vi "LogTest1.vi"() -> ()   [LabVIEW 2016]
panel:
  out "Experiment Description 2":T1
  out "date/time string":string
  out "current time":timestamp
  in  "file path":path
  in  "stop":bool
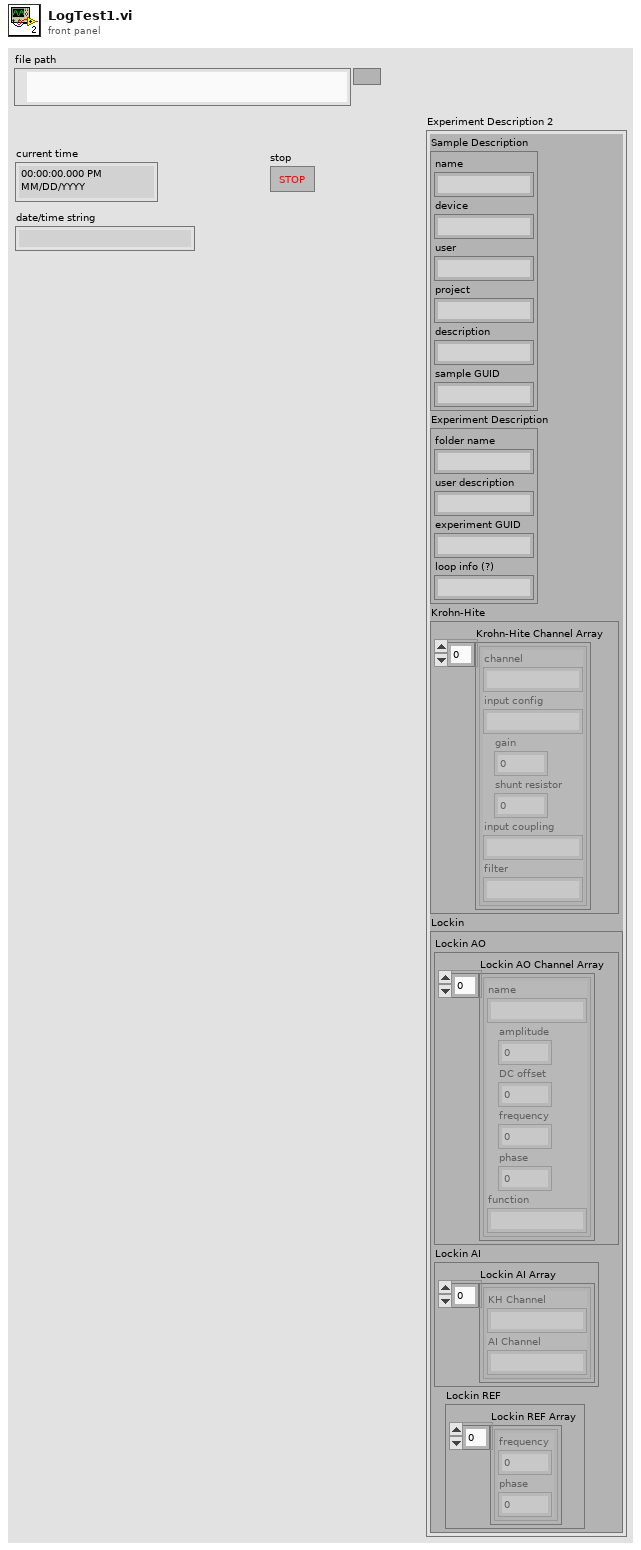
[diagram p1: front panel]
types:
  T1 = cluster{"Sample Description":cluster{"name":string, "device":string, "user":string, "project":string, "description":string, "sample GUID":string}, "Experiment Description":cluster{"folder name":string, "user description":string, "experiment GUID":string, "loop info (?)":string}, "Krohn-Hite":cluster{"Krohn-Hite Channel Array":cluster{"channel":string, "input config":string, "gain":i32, "shunt resistor":i32, "input coupling":string, "filter":string}[]}, "Lockin":cluster{"Lockin AO":cluster{"Lockin AO Channel Array":cluster{"name":string, "amplitude":dbl, "DC offset":dbl, "frequency":dbl, "phase":dbl, "function":string}[]}, "Lockin AI":cluster{"Lockin AI Array":cluster{"KH Channel":string, "AI Channel":string}[]}, "Lockin REF":cluster{"Lockin REF Array":cluster{"frequency":dbl, "phase":dbl}[]}}}
  T2 = enum16{"open", "open or create", "create or replace", "create", "open (read-only)"}
  T3 = cluster{"name":string, "device":string, "user":string, "project":string, "description":string, "sample GUID":string}
  T4 = cluster{"folder name":string, "user description":string, "experiment GUID":string, "loop info (?)":string}
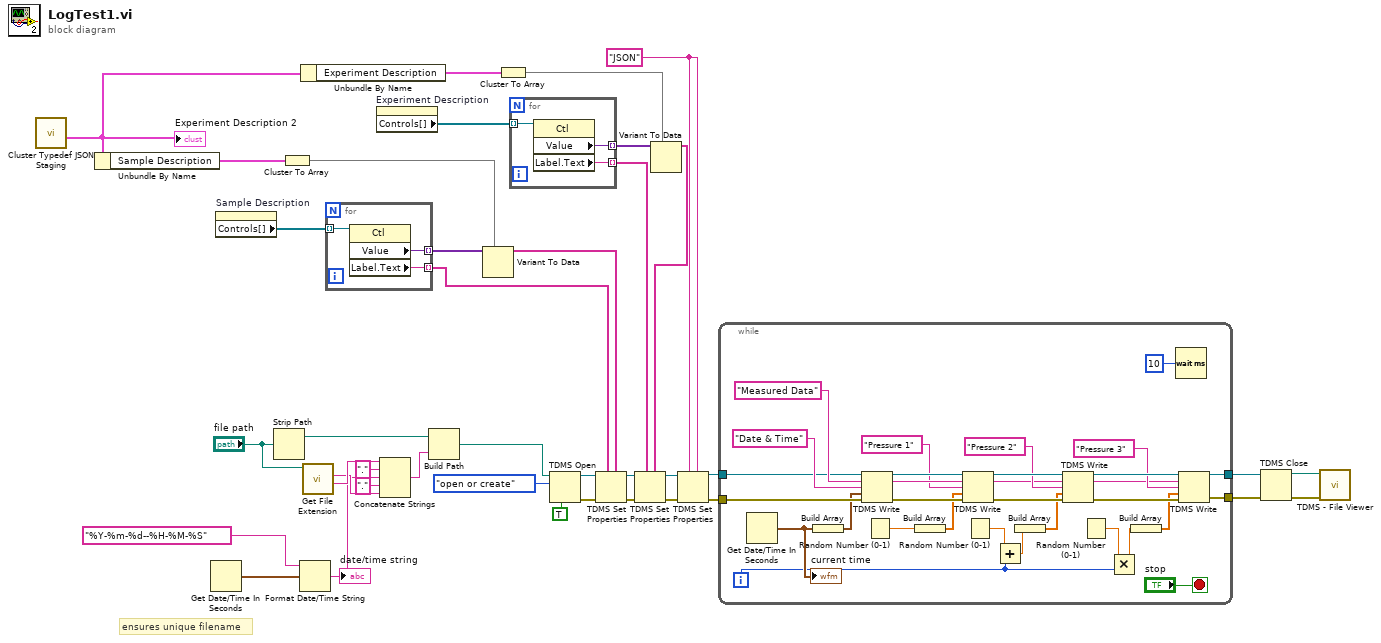
[diagram p0: block diagram]
diagram:
  w1 = "JSON"
  # "ensures unique filename"
  n1 = call "Cluster Typedef JSON Staging.vi"() -> ("Experiment Description 2"=w11:T1)  [unwired: 9 in, 2 out]
  "Experiment Description 2" <- w11
  n2 = Unbundle By Name(w11) -> ("Sample Description"=w16:T3)
  n3 = Get Date/Time In Seconds() -> (seconds since 1Jan1904=w35:timestamp)
  n4 = property on="Sample Description" class="Clust (strict)"() -> ("Controls[]"=w39:refnum<vi>[])  [unwired: 2 in, 2 out]
  n5 = Strip Path(path="file path") -> (stripped path=w19:path)  [unwired: 1 out]
  n6 = Cluster To Array(cluster=w16) -> (array=w37:string[])
  n7 = Format Date/Time String(time format string (%c)="%Y-%m-%d--%H-%M-%S", seconds (now)=w35) -> (date/time string=w31:string)  [unwired: 1 in]
  "date/time string" <- w31
  n8 = Unbundle By Name(w11) -> ("Experiment Description"=w15:T4)
  n9 = call <vilib>:"Get File Extension.vi"("file"="file path") -> ("filename without extension"=w33:string, "lowercase file extension"=w32:string)  [unwired: 6 in, 3 out]
  n10 = for {
    tunnel: w39 -> [w42] mode=indexing
    tunnel: [w41] -> w38 mode=indexing
    tunnel: [w40] -> w5 mode=indexing
    n11 = property class="Ctl"(reference=w42) -> ("Value"=w41:variant, "Label.Text"=w40:string)  [unwired: 1 in, 2 out]
  }
  n12 = property on="Experiment Description" class="Clust (strict)"() -> ("Controls[]"=w12:refnum<vi>[])  [unwired: 2 in, 2 out]
  n13 = Concatenate Strings(w33, "." ("string"), w31, "." ("string"), w32) -> (w18:string)
  n14 = Build Path(base path=w19, name or relative path=w18) -> (appended path=w17:path)
  n15 = Variant To Data(type=w37, Variant=w38) -> (data=w20:string[])  [unwired: 1 in, 1 out]
  n16 = Cluster To Array(cluster=w15) -> (array=w14:string[])
  n17 = for {
    tunnel: w12 -> [w45] mode=indexing
    tunnel: [w44] -> w13 mode=indexing
    tunnel: [w43] -> w4 mode=indexing
    n18 = property class="Ctl"(reference=w45) -> ("Value"=w44:variant, "Label.Text"=w43:string)  [unwired: 1 in, 2 out]
  }
  n19 = TDMS Open(6:TRUE ("disable buffering? (T)"), 10:T2."open or create" ("operation (0:open)"), 11:w17) -> (0:w22:errorcluster, 3:w21:refnum<k34>)  [unwired: 4 in]
  n20 = TDMS Set Properties(5:w20, 7:w5, 8:w22, 11:w21) -> (0:w9:errorcluster, 3:w7:refnum<k34>)  [unwired: 2 in, 2 out]
  n21 = Variant To Data(type=w14, Variant=w13) -> (data=w3:string[])  [unwired: 1 in, 1 out]
  n22 = TDMS Set Properties(5:w3, 7:w4, 8:w9, 11:w7) -> (0:w10:errorcluster, 3:w6:refnum<k34>)  [unwired: 2 in, 2 out]
  n23 = TDMS Set Properties(5:w1, 7:w1, 8:w10, 11:w6) -> (0:w8:errorcluster, 3:w2:refnum<k34>)  [unwired: 2 in, 2 out]
  n24 = while {
    tunnel: w8 -> [w73]
    tunnel: [w54] -> w24
    tunnel: [w53] -> w23
    tunnel: w2 -> [w46]
    i -> [w49]
    stop <- "stop" stop-if-true
    n25 = Get Date/Time In Seconds() -> (seconds since 1Jan1904=w52:timestamp)
    "current time" <- w52
    n26 = Build Array(w52) -> (w71:timestamp[])
    n27 = TDMS Write(0:w46, 5:"Measured Data" ("group name in (Untitled)"), 7:"Date & Time", 9:w71, 11:w73) -> (4:w70:refnum<k34>, 6:w68:string, 15:w69:errorcluster)  [unwired: 1 in, 1 out]
    n28 = Random Number (0-1)() -> (number: 0 to 1=w66:dbl)
    n29 = Build Array(w66) -> (w65:dbl[])
    n30 = TDMS Write(0:w70, 5:w68, 7:"Pressure 1", 9:w65, 11:w69) -> (4:w64:refnum<k34>, 6:w59:string, 15:w63:errorcluster)  [unwired: 1 in, 1 out]
    n31 = Random Number (0-1)() -> (number: 0 to 1=w48:dbl)
    n32 = Add(x=w48, y=w49) -> (x+y=w47:dbl)
    n33 = Build Array(w47) -> (w58:dbl[])
    n34 = TDMS Write(0:w64, 5:w59, 7:"Pressure 2", 9:w58, 11:w63) -> (4:w62:refnum<k34>, 6:w55:string, 15:w61:errorcluster)  [unwired: 1 in, 1 out]
    n35 = Random Number (0-1)() -> (number: 0 to 1=w51:dbl)
    n36 = Multiply(x=w51, y=w49) -> (x*y=w50:dbl)
    n37 = Build Array(w50) -> (w57:dbl[])
    n38 = Wait (ms)(milliseconds to wait=u32 10) -> ()  [unwired: 1 out]
    n39 = TDMS Write(0:w62, 5:w55, 7:"Pressure 3", 9:w57, 11:w61) -> (4:w54:refnum<k34>, 15:w53:errorcluster)  [unwired: 1 in, 2 out]
  }
  n40 = TDMS Close(8:w23, 11:w24) -> (0:w26:errorcluster, 3:w25:path)
  n41 = call <vilib>:"TDMS - File Viewer.vi"("error in (no error)"=w26, "file path"=w25) -> ()  [unwired: 4 in, 2 out]
